vi "Line Configuration Dialog.vi"(8 "error in":errorcluster, 9 "engine configuration in":refnum<class "engine configuration.lvclass">, 10 "tag bus configurable plugin module configuration":refnum<class "DAQmx Module Configuration.lvclass">, 11 "Line":T5={"channel"=refnum, "Physical Channel"="", "Measurement Type"=enum."Digital Input", "Parameters"={"Digital Config"={"Invert Lines?"=FALSE}, "Voltage Config"={"Maximum Value (V)"=5.0, "Minimum Value (V)"=-5.0, "in terminal configuration (V)"=-1, "out terminal configuration (V)"=-1}, "Current Config"={"Maximum Value (A)"=0.02, "Minimum Value (A)"=0.0, "shunt resistor location"=-1, "input terminal configuration (C)"=-1, "external shunt resistor value"=249.0}, "RTD Config"={"Maximum Value (°C)"=100.0, "Minimum Value (°C)"=0.0, "resistance configuration"=2, "r0"=100.0, "current excitation value"=0.0025, "rtd type"=10137, "current excitation source"=10167}, "Thermocouple Config"={"Minimum Value (C)"=0.0, "Maximum Value (C)"=100.0, "thermocouple type"=10072, "cjc source"=10116, "cjc value"=25.0}, "Strain Config"={"Maximum Value"=0.001, "Minimum Value"=-0.001, "bridge information"={"strain configuration"=10183, "lead wire resistance"=0.0, "initial bridge voltage"=0.0, "voltage excitation source"=10200, "voltage excitation value"=2.5}, "strain gage information"={"gage factor"=2.0, "nominal gage resistance"=350.0, "poisson ratio"=0.3}}}} {"Parameters"."Voltage Config"."out terminal configuration (V)" items=["Default"=-1, "RSE"=10083, "Differential"=10106, "Pseudodifferential"=12529]; "Parameters"."Voltage Config"."in terminal configuration (V)" items=["Default"=-1, "RSE"=10083, "NRSE"=10078, "Differential"=10106, "Pseudodifferential"=12529]; "Parameters"."Current Config"."shunt resistor location" items=["default"=-1, "Internal"=10200, "External"=10167]; "Parameters"."Current Config"."input terminal configuration (C)" items=["default"=-1, "RSE"=10083, "NRSE"=10078, "Differential"=10106, "Pseudodifferential"=12529]; "Parameters"."RTD Config"."resistance configuration" items=["2-Wire"=2, "3-Wire"=3, "4-Wire"=4]; "Parameters"."RTD Config"."rtd type" items=["Pt3750"=12481, "Pt3851"=10071, "Pt3911"=12482, "Pt3916"=10069, "Pt3920"=10053, "Pt3928"=12483, "Custom"=10137]; "Parameters"."RTD Config"."current excitation source" items=["Internal"=10200, "External"=10167, "None"=10230]; "Parameters"."Thermocouple Config"."thermocouple type" items=["J"=10072, "K"=10073, "N"=10077, "R"=10082, "S"=10085, "T"=10086, "B"=10047, "E"=10055]; "Parameters"."Thermocouple Config"."cjc source" items=["Built-In"=10200, "Constant Value"=10116, "Channel"=10113]; "Parameters"."Strain Config"."bridge information"."strain configuration" items=["Full Bridge I"=10183, "Full Bridge II"=10184, "Full Bridge III"=10185, "Half Bridge I"=10188, "Half Bridge II"=10189, "Quarter Bridge I"=10271, "Quarter Bridge II"=10272]; "Parameters"."Strain Config"."bridge information"."voltage excitation source" items=["Internal"=10200, "External"=10167, "None"=10230]}) -> (0 "error out":errorcluster, 1 "success":bool, 2 "changed":bool, 3 "Mappings out":T4={"Line"={"channel"=refnum, "Physical Channel"="", "Measurement Type"=enum."Digital Input", "Parameters"={"Digital Config"={"Invert Lines?"=FALSE}, "Voltage Config"={"Maximum Value (V)"=5.0, "Minimum Value (V)"=-5.0, "in terminal configuration (V)"=-1, "out terminal configuration (V)"=-1}, "Current Config"={"Maximum Value (A)"=0.02, "Minimum Value (A)"=0.0, "shunt resistor location"=-1, "input terminal configuration (C)"=-1, "external shunt resistor value"=249.0}, "RTD Config"={"Maximum Value (°C)"=100.0, "Minimum Value (°C)"=0.0, "resistance configuration"=2, "r0"=100.0, "current excitation value"=0.0025, "rtd type"=10137, "current excitation source"=10167}, "Thermocouple Config"={"Minimum Value (C)"=0.0, "Maximum Value (C)"=100.0, "thermocouple type"=10072, "cjc source"=10116, "cjc value"=25.0}, "Strain Config"={"Maximum Value"=0.001, "Minimum Value"=-0.001, "bridge information"={"strain configuration"=10183, "lead wire resistance"=0.0, "initial bridge voltage"=0.0, "voltage excitation source"=10200, "voltage excitation value"=2.5}, "strain gage information"={"gage factor"=2.0, "nominal gage resistance"=350.0, "poisson ratio"=0.3}}}}, "Maps"=[]} {"Line"."Parameters"."Voltage Config"."out terminal configuration (V)" items=["Default"=-1, "RSE"=10083, "Differential"=10106, "Pseudodifferential"=12529]; "Line"."Parameters"."Voltage Config"."in terminal configuration (V)" items=["Default"=-1, "RSE"=10083, "NRSE"=10078, "Differential"=10106, "Pseudodifferential"=12529]; "Line"."Parameters"."Current Config"."shunt resistor location" items=["default"=-1, "Internal"=10200, "External"=10167]; "Line"."Parameters"."Current Config"."input terminal configuration (C)" items=["default"=-1, "RSE"=10083, "NRSE"=10078, "Differential"=10106, "Pseudodifferential"=12529]; "Line"."Parameters"."RTD Config"."resistance configuration" items=["2-Wire"=2, "3-Wire"=3, "4-Wire"=4]; "Line"."Parameters"."RTD Config"."rtd type" items=["Pt3750"=12481, "Pt3851"=10071, "Pt3911"=12482, "Pt3916"=10069, "Pt3920"=10053, "Pt3928"=12483, "Custom"=10137]; "Line"."Parameters"."RTD Config"."current excitation source" items=["Internal"=10200, "External"=10167, "None"=10230]; "Line"."Parameters"."Thermocouple Config"."thermocouple type" items=["J"=10072, "K"=10073, "N"=10077, "R"=10082, "S"=10085, "T"=10086, "B"=10047, "E"=10055]; "Line"."Parameters"."Thermocouple Config"."cjc source" items=["Built-In"=10200, "Constant Value"=10116, "Channel"=10113]; "Line"."Parameters"."Strain Config"."bridge information"."strain configuration" items=["Full Bridge I"=10183, "Full Bridge II"=10184, "Full Bridge III"=10185, "Half Bridge I"=10188, "Half Bridge II"=10189, "Quarter Bridge I"=10271, "Quarter Bridge II"=10272]; "Line"."Parameters"."Strain Config"."bridge information"."voltage excitation source" items=["Internal"=10200, "External"=10167, "None"=10230]})   [LabVIEW 2014, in "DAQmx Module Editor Node.lvclass"]
doc: "A dialog for allowing a user to specify the values of a new line."
uses:
  DAQmx Module Editor Node.lvclass
  module/configuration/Line.ctl
  <vilib>/NI/Tag Bus Module Framework/channel/TBM channel.lvclass
  module/configuration/Measurement Type.ctl
  module/configuration/Parameters.ctl
  Mappings.ctl
  Map.ctl
  <vilib>/NI/Module Execution Interface/Engine Configuration/engine configuration.lvclass
  module/configuration/DAQmx Module Configuration.lvclass
  <vilib>/NI/Tag Bus/tag/tag descriptor.lvclass/tag descriptor.ctl
  <vilib>/NI/Configuration Framework/serializable configuration/NISE_CEF_serializable configuration.lvclass/NISE_CEF_serializable configuration.ctl
  <vilib>/NI/Tag Bus Module Framework/channel/TBM channel.lvclass/TBM channel.ctl
  <vilib>/NI/Tag Bus/tag/write metadata.vi
  <vilib>/NI/Tag Bus/tag/write tag name.vi
  <vilib>/NI/Tag Bus/tag/write data type.vi
  <vilib>/NI/Tag Bus Module Framework/channel/Write channel classification.vi
  <vilib>/NI/Configuration Framework/serializable configuration/Read UID.vi
  <vilib>/NI/Tag Bus/tag/read metadata.vi
  <vilib>/Utility/LVClass/Get LV Class Name.vi
  <vilib>/NI/Configuration Framework/error generator/NISE_error generator.vi
  <vilib>/NI/Tag Bus/tag/tag descriptor.lvclass
  <vilib>/NI/DCAF UI Toolkit/Controls/DCAF UI Elements.lvlib
panel:
  in  "DAQmx Physical Channel":tag
  out "Tab Control":T1(tab)
  in  "Invert Lines?":bool
  in  "out terminal configuration (V)":i32(ring)=-1 items=["Default"=-1, "RSE"=10083, "Differential"=10106, "Pseudodifferential"=12529]
  in  "in terminal configuration (V)":i32(ring)=-1 items=["Default"=-1, "RSE"=10083, "NRSE"=10078, "Differential"=10106, "Pseudodifferential"=12529]
  in  "Maximum Value (V)":dbl=5.0 format="%0.2f"
  in  "Minimum Value (V)":dbl=-5.0 format="%0.2f"
  in  "input terminal configuration (C)":i32(ring)=-1 items=["default"=-1, "RSE"=10083, "NRSE"=10078, "Differential"=10106, "Pseudodifferential"=12529]
  in  "shunt resistor location":i32(ring)=-1 items=["default"=-1, "Internal"=10200, "External"=10167]
  in  "external shunt resistor value":dbl=249.0 format="%0.2f"
  in  "Maximum Value (A)":dbl=0.02 format="%0.5f"
  in  "Minimum Value (A)":dbl format="%0.5f"
  in  "r0":dbl=100.0 format="%0.2f"
  in  "resistance configuration":i32(ring)=2 items=["2-Wire"=2, "3-Wire"=3, "4-Wire"=4]
  in  "Maximum Value (°C)":dbl=100.0 format="%0.2f"
  in  "Minimum Value (°C)":dbl format="%0.2f"
  in  "rtd type":i32(ring)=12481 items=["Pt3750"=12481, "Pt3851"=10071, "Pt3911"=12482, "Pt3916"=10069, "Pt3920"=10053, "Pt3928"=12483, "Custom"=10137]
  in  "current excitation value":dbl=0.0025 format="%0.5f"
  in  "current excitation source":i32(ring)=10167 items=["Internal"=10200, "External"=10167, "None"=10230]
  in  "strain gage information":T2={"gage factor"=2.0, "nominal gage resistance"=350.0, "poisson ratio"=0.3} {"poisson ratio" format="%0.2f"; "nominal gage resistance" format="%0.2f"; "gage factor" format="%0.2f"}
  in  "bridge information":T3={"strain configuration"=10183, "lead wire resistance"=0.0, "initial bridge voltage"=0.0, "voltage excitation source"=10200, "voltage excitation value"=2.5} {"initial bridge voltage" format="%0.2f"; "voltage excitation source" items=["Internal"=10200, "External"=10167, "None"=10230]; "voltage excitation value" format="%0.2f"; "lead wire resistance" format="%0.2f"; "strain configuration" items=["Full Bridge I"=10183, "Full Bridge II"=10184, "Full Bridge III"=10185, "Half Bridge I"=10188, "Half Bridge II"=10189, "Quarter Bridge I"=10271, "Quarter Bridge II"=10272]}
  in  "Minimum Value":dbl=-0.001 format="%0.7f"
  in  "Maximum Value":dbl=0.001 format="%0.7f"
  in  "cjc value":dbl=25.0 format="%0.2f"
  in  "thermocouple type":i32(ring)=10072 items=["J"=10072, "K"=10073, "N"=10077, "R"=10082, "S"=10085, "T"=10086, "B"=10047, "E"=10055]
  in  "Maximum Value (C)":dbl=100.0 format="%0.2f"
  in  "Minimum Value (C)":dbl format="%0.2f"
  in  "cjc source":i32(ring)=10116 items=["Built-In"=10200, "Constant Value"=10116, "Channel"=10113]
  in  "Measurement Type":i32(listbox)
  out "errors":string
  in  "Tag":i32(listbox)
  in  "Description":string
  in  "cancel":bool
  in  "ok":bool
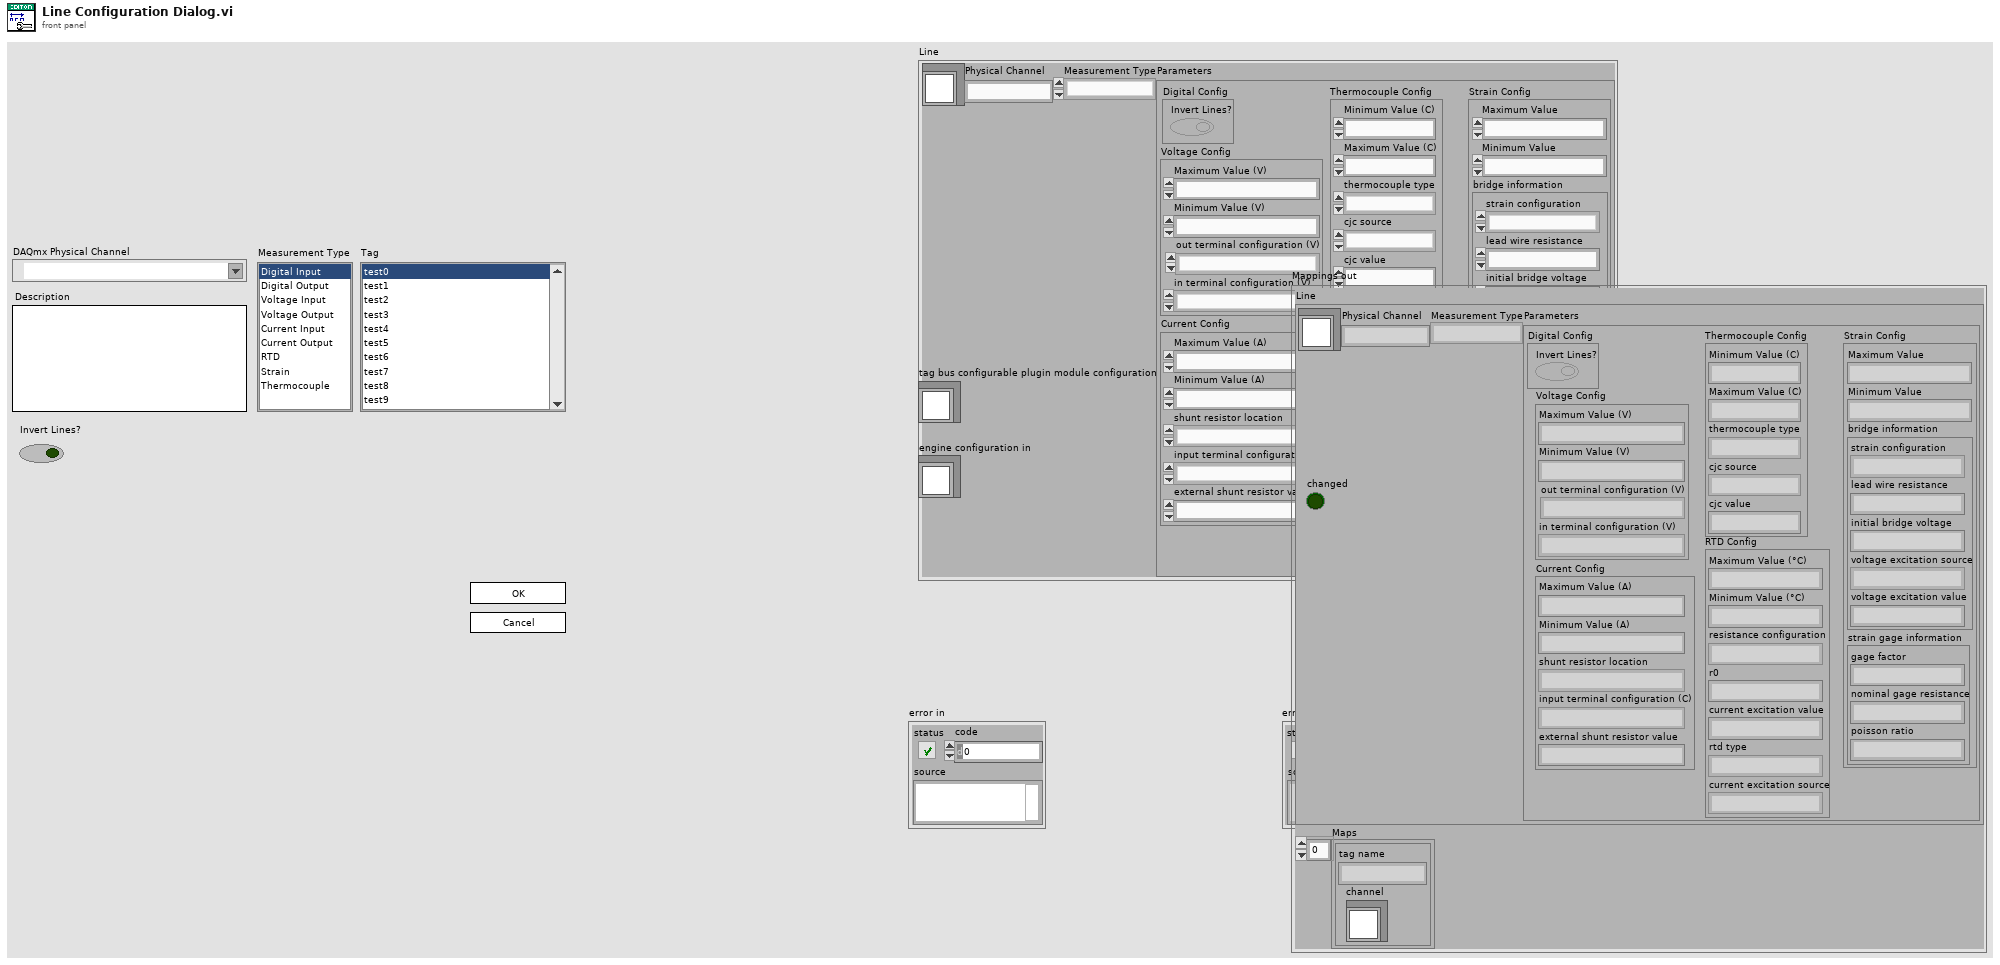
[diagram p1: front panel]
types:
  T1 = enum32{"Digital", "Voltage", "Current", "RTD", "Strain", "Thermocouple"}
  T2 = cluster{"gage factor":dbl, "nominal gage resistance":dbl, "poisson ratio":dbl}
  T3 = cluster{"strain configuration":i32, "lead wire resistance":dbl, "initial bridge voltage":dbl, "voltage excitation source":i32, "voltage excitation value":dbl}
  T4 = typedef "DAQmx Module Editor Node.lvclass/Mappings.ctl" = cluster{"Line":T5, "Maps":T8[]}
  T5 = typedef "DAQmx Module Configuration.lvclass/Line.ctl" = cluster{"channel":refnum<class "TBM channel.lvclass">, "Physical Channel":string, "Measurement Type":T6, "Parameters":T7}
  T6 = typedef "DAQmx Module Configuration.lvclass/Measurement Type.ctl" = enum16{"Digital Input", "Digital Output", "Voltage Input", "Voltage Output", "Current Input", "Current Output", "RTD", "Thermocouple", "Strain"}
  T7 = typedef "DAQmx Module Configuration.lvclass/Parameters.ctl" = cluster{"Digital Config":cluster{"Invert Lines?":bool}, "Voltage Config":cluster{"Maximum Value (V)":dbl, "Minimum Value (V)":dbl, "in terminal configuration (V)":i32, "out terminal configuration (V)":i32}, "Current Config":cluster{"Maximum Value (A)":dbl, "Minimum Value (A)":dbl, "shunt resistor location":i32, "input terminal configuration (C)":i32, "external shunt resistor value":dbl}, "RTD Config":cluster{"Maximum Value (°C)":dbl, "Minimum Value (°C)":dbl, "resistance configuration":i32, "r0":dbl, "current excitation value":dbl, "rtd type":i32, "current excitation source":i32}, "Thermocouple Config":cluster{"Minimum Value (C)":dbl, "Maximum Value (C)":dbl, "thermocouple type":i32, "cjc source":i32, "cjc value":dbl}, "Strain Config":cluster{"Maximum Value":dbl, "Minimum Value":dbl, "bridge information":cluster{"strain configuration":i32, "lead wire resistance":dbl, "initial bridge voltage":dbl, "voltage excitation source":i32, "voltage excitation value":dbl}, "strain gage information":cluster{"gage factor":dbl, "nominal gage resistance":dbl, "poisson ratio":dbl}}}
  T8 = typedef "Daqmx Module editor node.lvclass/Map.ctl" = cluster{"channel":refnum<class "TBM channel.lvclass">, "tag name":string}
  T9 = typedef "Daqmx Module configuration.lvclass/Measurement Type.ctl" = enum16{"Digital Input", "Digital Output", "Voltage Input", "Voltage Output", "Current Input", "Current Output", "RTD", "Thermocouple", "Strain"}
  T10 = enum8{"Enabled", "Disabled", "Disabled and Grayed Out"}
  T11 = typedef "TBM channel.lvclass/channel classification.ctl" = enum16{"input data", "output data", "processing parameter", "processing result"}
  T12 = typedef "tag bus.lvlib/tag descriptor.lvclass/Data Type.ctl" = enum16{"Double", "Single", "I64", "I32", "I16", "I8", "U64", "U32", "U16", "U8", "Boolean", "String", "Array of Double", "Array of Single", "Array of I64", "Array of I32", "Array of I16", "Array of I8", "Array of U64", "Array of U32", "Array of U16", "Array of U8", "Array of Boolean", "Array of String"}
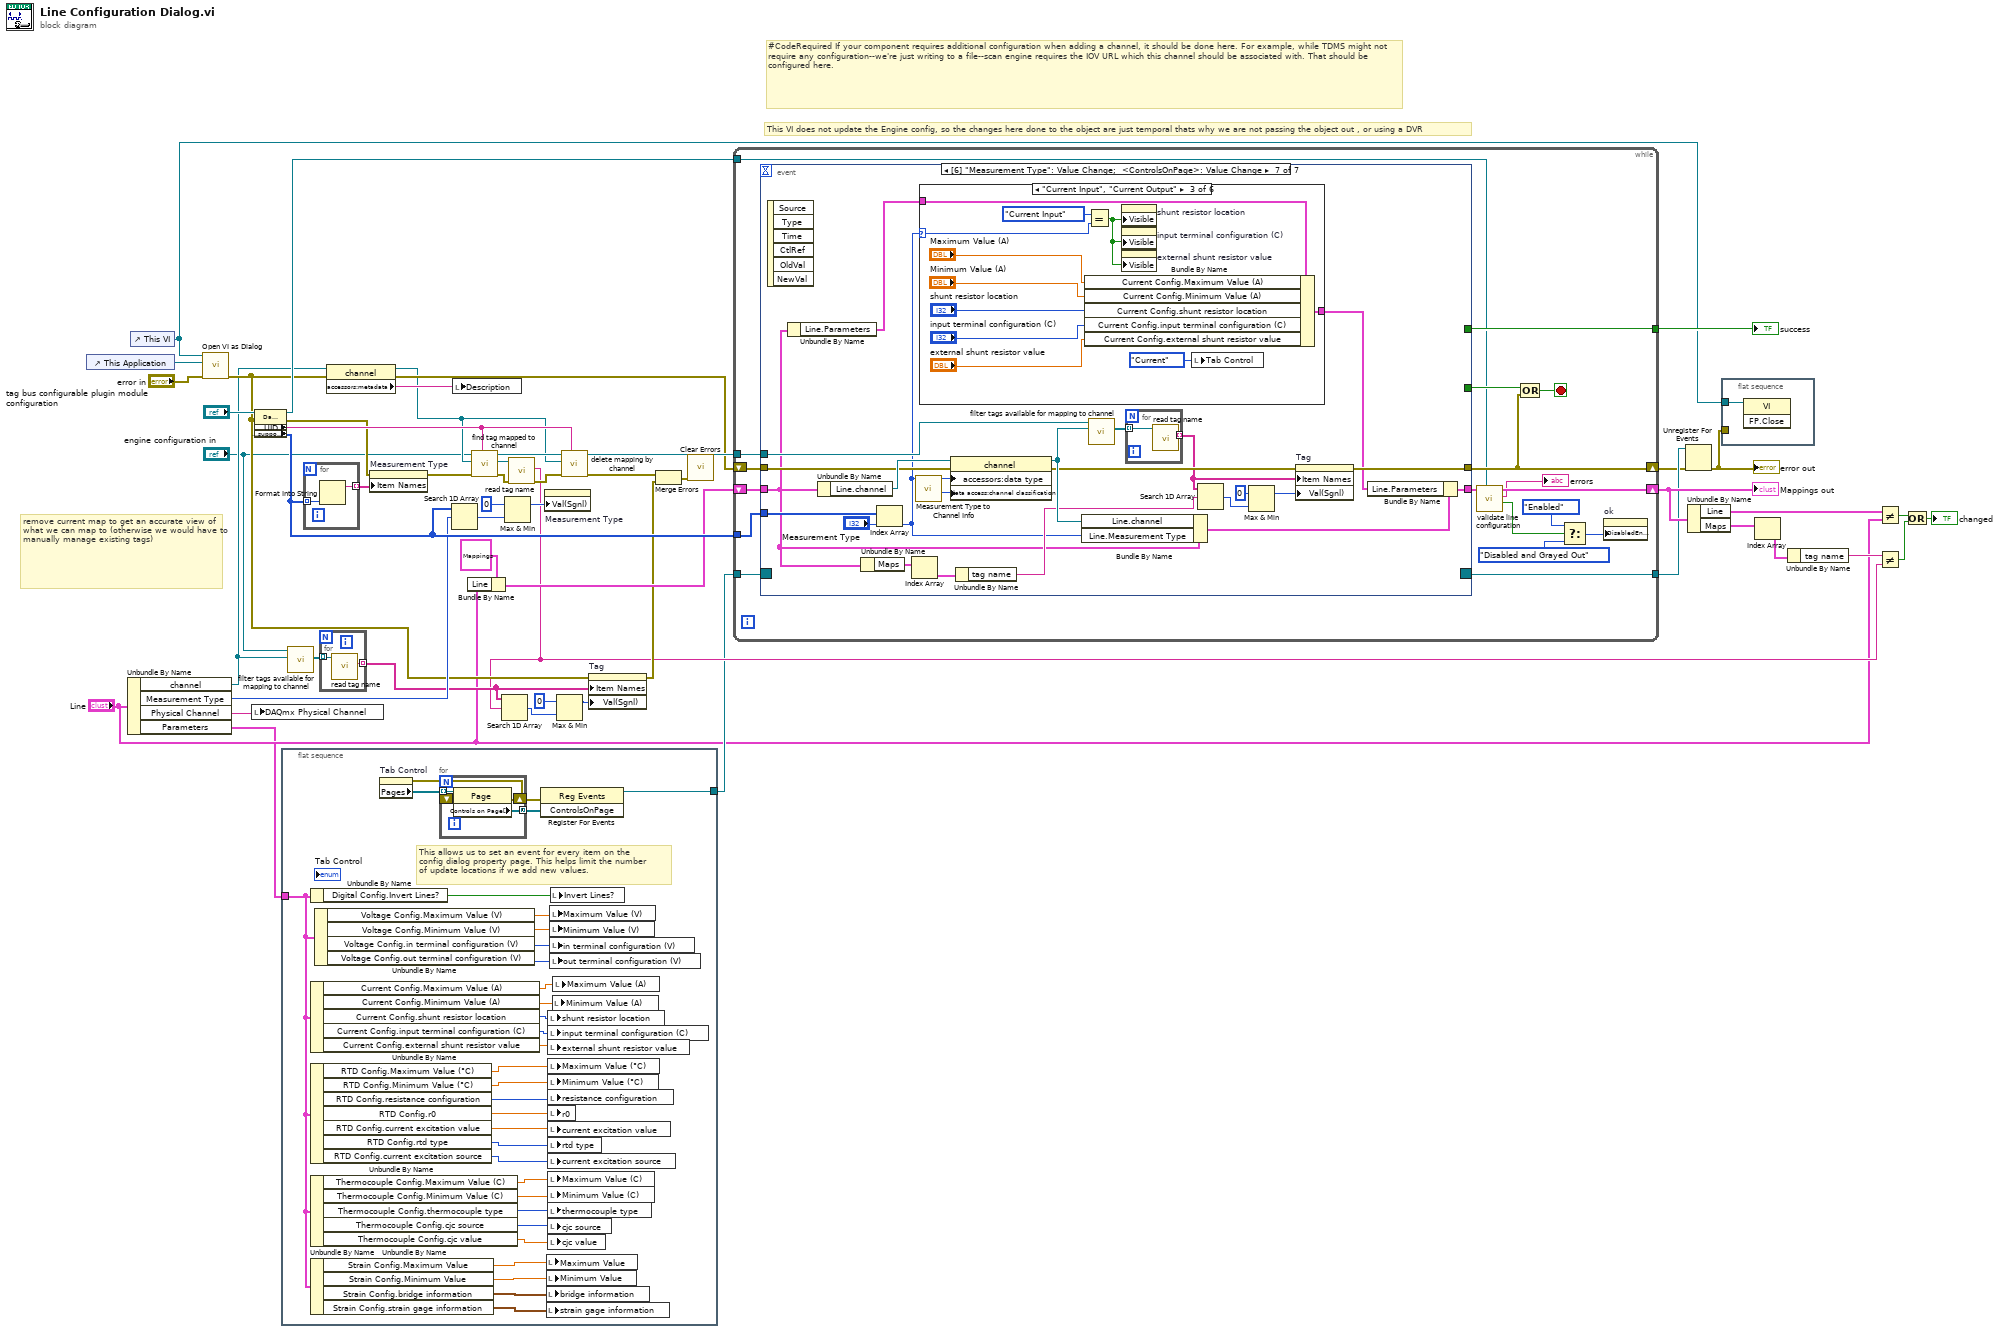
[diagram p0: block diagram]
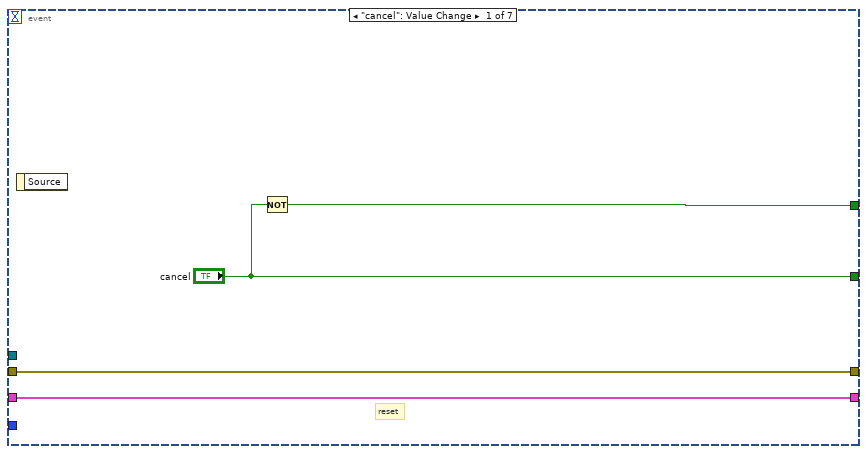
[diagram p2: hidden frame]
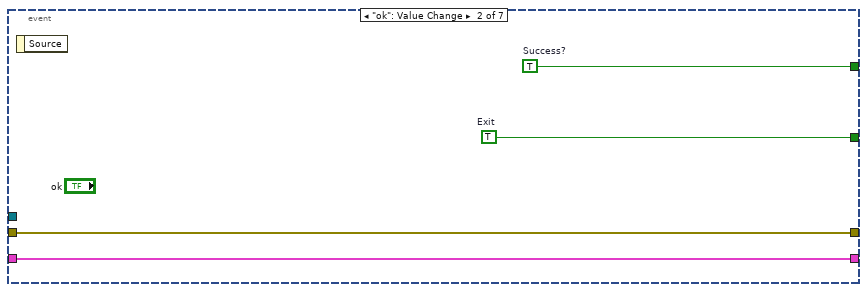
[diagram p3: hidden frame]
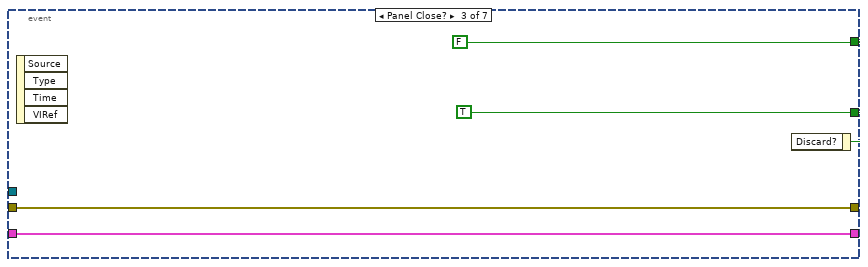
[diagram p4: hidden frame]
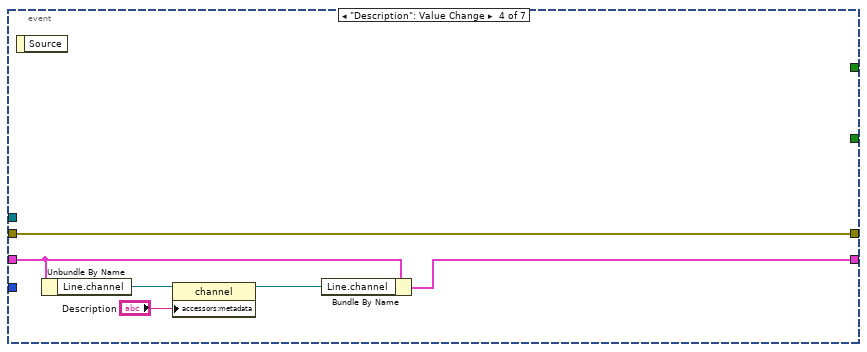
[diagram p5: hidden frame]
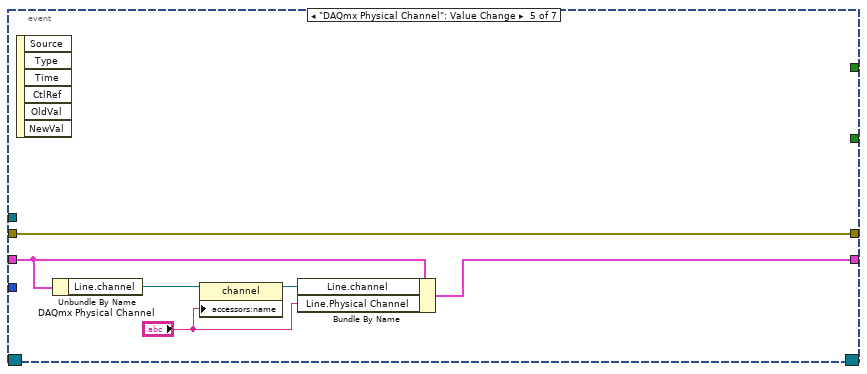
[diagram p6: hidden frame]
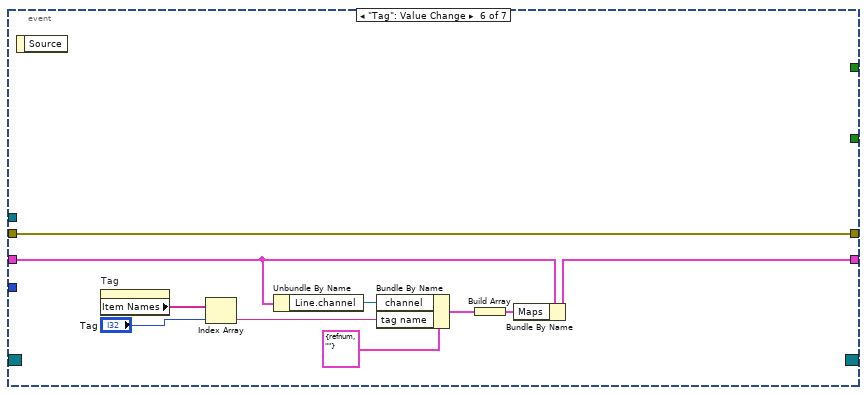
[diagram p7: hidden frame]
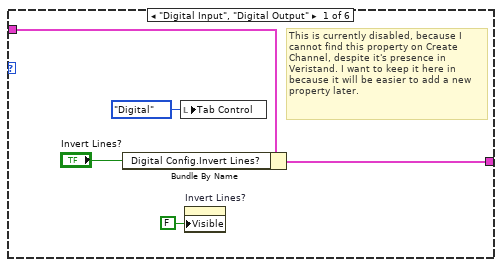
[diagram p8: hidden frame]
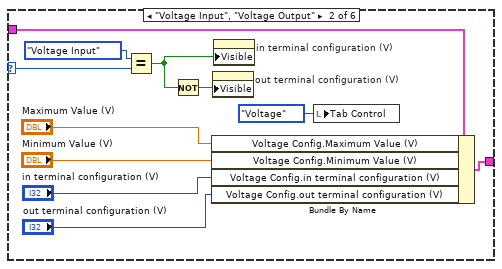
[diagram p9: hidden frame]
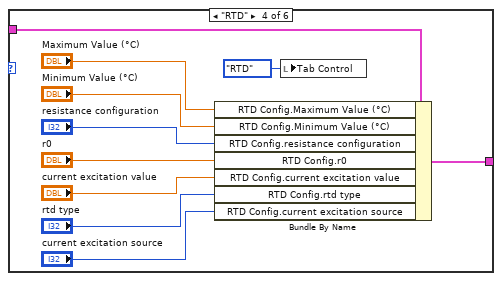
[diagram p10: hidden frame]
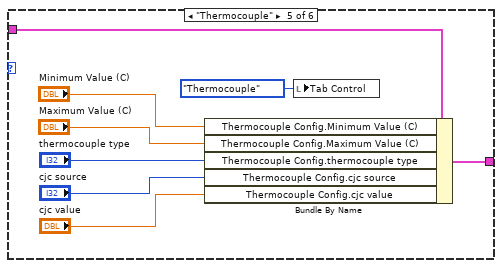
[diagram p11: hidden frame]
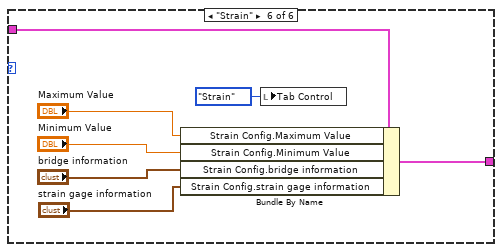
[diagram p12: hidden frame]
diagram:
  # "This VI does not update the Engine config, so the changes here done to the object are just temporal thats why we are not passing the object out , or using a DVR"
  # "remove current map to get an accurate view of what we can map to (otherwise we would have to manually manage existing tags)"
  # "#CodeRequired If your component requires additional configuration when adding a channel, it should be done here. For example, while TDMS might not require any configuration--we're just writing to a file--scan engine requires the IOV URL which this channel should be associated with. That should be configured here."
  n1 = control-ref of="This Application"() -> (w45:refnum<vi>)
  n2 = Unbundle By Name("Line") -> ("channel"=w17:refnum<class "TBM channel.lvclass">, "Measurement Type"=w22:T6, "Physical Channel"=w21:string, "Parameters"=w5:T7)
  n3 = control-ref of="This VI"() -> (w29:refnum<vi>)
  n4 = call <vilib>:"Open VI as Dialog.vi"("error in (no error)"="error in", "This Application"=w45, "VI in"=w29) -> ("error out"=w18:errorcluster)  [unwired: 8 in]
  n5 = local write "DAQmx Physical Channel"(w21) -> ()
  n6 = property class="Daqmx Module configuration"(reference="tag bus configurable plugin module configuration", error in=w18) -> (reference out=w40:refnum<class "DAQmx Module Configuration.lvclass">, error out=w27:errorcluster, "Properties:UID"=w43:string, "Customize:Properties:supported measurement types"=w23:T9[])
  n7 = flat-sequence {
    tunnel: [w84] -> w7
    tunnel: w5 -> [w58]
    frame #0 {
      # "This allows us to set an event for every item on the \nconfig dialog property page. This helps limit the number \nof update locations if we add new values."
      n8 = Unbundle By Name(w58) -> ("Digital Config.Invert Lines?"=w79:bool)
      n9 = Unbundle By Name(w58) -> ("Current Config.Maximum Value (A)"=w71:dbl, "Current Config.Minimum Value (A)"=w72:dbl, "Current Config.shunt resistor location"=w74:i32, "Current Config.input terminal configuration (C)"=w83:i32, "Current Config.external shunt resistor value"=w73:dbl)
      n10 = Unbundle By Name(w58) -> ("RTD Config.Maximum Value (°C)"=w70:dbl, "RTD Config.Minimum Value (°C)"=w69:dbl, "RTD Config.resistance configuration"=w68:i32, "RTD Config.r0"=w67:dbl, "RTD Config.current excitation value"=w66:dbl, "RTD Config.rtd type"=w65:i32, "RTD Config.current excitation source"=w64:i32)
      n11 = Unbundle By Name(w58) -> ("Thermocouple Config.Maximum Value (C)"=w61:dbl, "Thermocouple Config.Minimum Value (C)"=w62:dbl, "Thermocouple Config.thermocouple type"=w63:i32, "Thermocouple Config.cjc source"=w60:i32, "Thermocouple Config.cjc value"=w59:dbl)
      n12 = Unbundle By Name(w58) -> ("Strain Config.Maximum Value"=w75:dbl, "Strain Config.Minimum Value"=w76:dbl, "Strain Config.bridge information"=w77:T3, "Strain Config.strain gage information"=w78:T2)
      n13 = Unbundle By Name(w58) -> ("Voltage Config.Maximum Value (V)"=w82:dbl, "Voltage Config.Minimum Value (V)"=w81:dbl, "Voltage Config.in terminal configuration (V)"=w80:i32, "Voltage Config.out terminal configuration (V)"=w57:i32)
      n14 = property on="Tab Control" class="TabCtl (strict)"() -> (error out=w55:errorcluster, "Pages"=w56:refnum<vi>[])  [unwired: 2 in, 1 out]
      n15 = for {
        tunnel: w56 -> [w88] mode=indexing
        tunnel: [w85] -> w53 mode=concatenating
        shift-right: [w86] -> w54
        shift-left: w55 -> [w87]
        n16 = property class="Page"(reference=w88, error in=w87) -> (error out=w86:errorcluster, "Controls on Page[]"=w85:refnum<vi>[])  [unwired: 1 out]
      }
      n17 = register-events(error in=w54, w53) -> (reference out=w84:refnum<event-registration>)  [unwired: 1 in, 1 out]
      n18 = local write "Maximum Value"(w75) -> ()
      n19 = local write "Minimum Value"(w76) -> ()
      n20 = local write "bridge information"(w77) -> ()
      n21 = local write "strain gage information"(w78) -> ()
      n22 = local write "shunt resistor location"(w74) -> ()
      n23 = local write "input terminal configuration (C)"(w83) -> ()
      n24 = local write "external shunt resistor value"(w73) -> ()
      n25 = local write "Maximum Value (°C)"(w70) -> ()
      n26 = local write "Minimum Value (°C)"(w69) -> ()
      n27 = local write "resistance configuration"(w68) -> ()
      n28 = local write "r0"(w67) -> ()
      n29 = local write "current excitation value"(w66) -> ()
      n30 = local write "rtd type"(w65) -> ()
      n31 = local write "current excitation source"(w64) -> ()
      n32 = local write "Maximum Value (C)"(w61) -> ()
      n33 = local write "Minimum Value (C)"(w62) -> ()
      n34 = local write "thermocouple type"(w63) -> ()
      n35 = local write "cjc source"(w60) -> ()
      n36 = local write "cjc value"(w59) -> ()
      n37 = local write "Maximum Value (V)"(w82) -> ()
      n38 = local write "Minimum Value (V)"(w81) -> ()
      n39 = local write "in terminal configuration (V)"(w80) -> ()
      n40 = local write "out terminal configuration (V)"(w57) -> ()
      n41 = local write "Invert Lines?"(w79) -> ()
      n42 = local write "Minimum Value (A)"(w72) -> ()
      n43 = local write "Maximum Value (A)"(w71) -> ()
    }
  }
  n44 = call-dynamic "filter tags available for mapping to channel.vi"("channel to map to"=w17, "engine configuration in"="engine configuration in") -> ("filtered tags"=w19:refnum<class "tag descriptor.lvclass">[])  [unwired: 8 in, 1 out]
  n45 = for {
    tunnel: w23 -> [w90] mode=indexing
    tunnel: [w89] -> w28 mode=indexing
    n46 = Format Into String(w90) -> (resulting string=w89:string)  [unwired: 3 in, 1 out]
  }
  n47 = for {
    tunnel: w19 -> [w92] mode=indexing
    tunnel: [w91] -> w15 mode=indexing
    n48 = call <vilib>:"read tag name.vi"("system tag in"=w92) -> ("name"=w91:string)  [unwired: 8 in, 2 out]
  }
  n49 = property class="channel"(reference=w17, error in=w18) -> (reference out=w39:refnum<class "TBM channel.lvclass">, error out=w41:errorcluster, "accessors:metadata"=w50:string)
  n50 = property on="Measurement Type" class="LstBox (strict)"(error in=w27, "Item Names"=w28) -> (error out=w1:errorcluster)  [unwired: 1 in, 1 out]
  n51 = Search 1D Array(1D array=w23, element=w22) -> (index of element=w24:i32)  [unwired: 1 in]
  n52 = local write "Description"(w50) -> ()
  n53 = Bundle By Name(cluster=T4 {"Line"={"channel"=refnum, "Physical Channel"="", "Measurement Type"=enum."Digital Input", "Parameters"={"Digital Config"={"Invert Lines?"=FALSE}, "Voltage Config"={"Maximum Value (V)"=5.0, "Minimum Value (V)"=-5.0, "in terminal configuration (V)"=-1, "out terminal configuration (V)"=-1}, "Current Config"={"Maximum Value (A)"=0.02, "Minimum Value (A)"=0.0, "shunt resistor location"=-1, "input terminal configuration (C)"=-1, "external shunt resistor value"=249.0}, "RTD Config"={"Maximum Value (°C)"=100.0, "Minimum Value (°C)"=0.0, "resistance configuration"=2, "r0"=100.0, "current excitation value"=0.0025, "rtd type"=10137, "current excitation source"=10167}, "Thermocouple Config"={"Minimum Value (C)"=0.0, "Maximum Value (C)"=100.0, "thermocouple type"=10072, "cjc source"=10116, "cjc value"=25.0}, "Strain Config"={"Maximum Value"=0.001, "Minimum Value"=-0.001, "bridge information"={"strain configuration"=10183, "lead wire resistance"=0.0, "initial bridge voltage"=0.0, "voltage excitation source"=10200, "voltage excitation value"=2.5}, "strain gage information"={"gage factor"=2.0, "nominal gage resistance"=350.0, "poisson ratio"=0.3}}}}, "Maps"=[]} ("Mappings out"), "Line"="Line") -> (w20:T4)
  n54 = call <vilib>:"find tag mapped to channel.vi"("owner"=w43, "error in"=w1, "channel"=w39, "engine configuration in"="engine configuration in") -> ("error out"=w37:errorcluster, "tag"=w38:refnum<class "tag descriptor.lvclass">, "engine configuration out"=w42:refnum<class "engine configuration.lvclass">)  [unwired: 5 in]
  n55 = Max & Min(x=0 ("f"), y=w24) -> (max(x,y)=w26:i32)  [unwired: 1 out]
  n56 = call <vilib>:"read tag name.vi"("error in"=w37, "system tag in"=w38) -> ("error out"=w36:errorcluster, "name"=w9:string)  [unwired: 7 in, 1 out]
  n57 = Search 1D Array(1D array=w15, element=w9) -> (index of element=w10:i32)  [unwired: 1 in]
  n58 = property on="Measurement Type" class="LstBox (strict)"("Val(Sgnl)"=w26) -> ()  [unwired: 2 in, 2 out]
  n59 = Max & Min(x=0 ("f"), y=w10) -> (max(x,y)=w8:i32)  [unwired: 1 out]
  n60 = call <vilib>:"delete mapping by channel.vi"("owner ID"=w43, "error in"=w36, "channel"=w39, "engine configuration in"=w42) -> ("error out"=w14:errorcluster, "engine configuration out"=w51:refnum<class "engine configuration.lvclass">)  [unwired: 6 in]
  n61 = property on="Tag" class="LstBox (strict)"(error in=w18, "Item Names"=w15, "Val(Sgnl)"=w8) -> (error out=w13:errorcluster)  [unwired: 1 in, 1 out]
  n62 = Merge Errors(w14, w13) -> (w12:errorcluster)
  n63 = call <vilib>:"Clear Errors.vi"("error in (no error)"=w12) -> ()  [unwired: 5 in, 2 out]
  n64 = while {
    shift-right: [w102] -> w3
    shift-left: w41 -> [w109]
    tunnel: [w108] -> w52
    shift-right: [w103] -> w46
    shift-left: w20 -> [w105]
    tunnel: w51 -> [w110]
    tunnel: w40 -> [w94]
    tunnel: w23 -> [w96]
    tunnel: w7 -> [w95]
    tunnel: [w93] -> w4
    stop <- w106 stop-if-true
    n65 = event shown="[6] \"Measurement Type\": Value Change;  <ControlsOnPage>: Value Change" {
      selector: w95 -> [_ _ _ _ _ _ _]
      dyn-events: [_ _ _ _ _ _ _] -> w93
      timeout: _ -> [_ _ _ _ _ _ _]
      tunnel: w110 -> [_ _ _ _ _ _ w159]
      tunnel: w109 -> [w114 w118 w122 w128 w134 w144 w165]
      tunnel: [w114 w118 w122 w128 w134 w144 w163] -> w102
      tunnel: [w113 w115 FALSE _ _ _ _] -> w108
      tunnel: ["cancel" w116 w120 _ _ _ _] -> w107
      tunnel: w105 -> [w111 w117 w119 w126 w132 w139 w151]
      tunnel: [w111 w117 w119 w127 w133 w136 w149] -> w104
      tunnel: w96 -> [_ _ _ _ _ _ w157]
      event "cancel": Value Change {
        # "reset"
        n66 = event-data() -> ()  [unwired: 1 in, 1 out]
        n67 = Not(x="cancel") -> (.not. x?=w113:bool)
      }
      event "ok": Value Change {
        w115 = TRUE  # Success?
        w116 = TRUE  # Exit
        n68 = event-data() -> ()  [unwired: 1 in, 1 out]
      }
      event Panel Close? {
        w120 = TRUE ("cancel")
        n69 = event-data() -> ()  [unwired: 1 in, 4 out]
        n70 = event-data("Discard?"=w120) -> ()  [unwired: 1 in, 1 out]
      }
      event "Description": Value Change {
        n71 = event-data() -> ()  [unwired: 1 in, 1 out]
        n72 = Unbundle By Name(w126) -> ("Line.channel"=w125:refnum<class "TBM channel.lvclass">)
        n73 = property class="channel"(reference=w125, "accessors:metadata"="Description") -> (reference out=w124:refnum<class "TBM channel.lvclass">)  [unwired: 1 in, 1 out]
        n74 = Bundle By Name(cluster=w126, "Line.channel"=w124) -> (w127:T4)
      }
      event "DAQmx Physical Channel": Value Change {
        n75 = event-data() -> ()  [unwired: 1 in, 6 out]
        n76 = Unbundle By Name(w132) -> ("Line.channel"=w131:refnum<class "TBM channel.lvclass">)
        n77 = property class="channel"(reference=w131, "accessors:name"="DAQmx Physical Channel") -> (reference out=w130:refnum<class "TBM channel.lvclass">)  [unwired: 1 in, 1 out]
        n78 = Bundle By Name(cluster=w132, "Line.channel"=w130, "Line.Physical Channel"="DAQmx Physical Channel") -> (w133:T4)
      }
      event "Tag": Value Change {
        n79 = event-data() -> ()  [unwired: 1 in, 1 out]
        n80 = property on="Tag" class="LstBox (strict)"() -> ("Item Names"=w142:string[])  [unwired: 2 in, 2 out]
        n81 = Index Array(array=w142, index="Tag") -> (element=w135:string)
        n82 = Unbundle By Name(w139) -> ("Line.channel"=w140:refnum<class "TBM channel.lvclass">)
        n83 = Bundle By Name(cluster=T8 {"channel"=refnum, "tag name"=""} ("Map"), "channel"=w140, "tag name"=w135) -> (w138:T8)
        n84 = Build Array(w138) -> (w137:T8[])
        n85 = Bundle By Name(cluster=w139, "Maps"=w137) -> (w136:T4)
      }
      event "Measurement Type": Value Change {
        n86 = event-data() -> ()  [unwired: 1 in, 6 out]
        n87 = Unbundle By Name(w151) -> ("Line.Parameters"=w148:T7)
        n88 = Unbundle By Name(w151) -> ("Line.channel"=w168:refnum<class "TBM channel.lvclass">)
        n89 = Unbundle By Name(w151) -> ("Maps"=w161:T8[])
        n90 = Index Array(array=w157, index="Measurement Type") -> (element=w152:T9)
        n91 = Index Array(array=w161) -> (element=w160:T8)  [unwired: 1 in]
        n92 = call "Measurement Type to Channel Info.vi"("Measurement Type"=w152) -> ("channel classification"=w145:T11, "Data Type"=w146:T12)  [unwired: 8 in]
        n93 = case shown="\"Current Input\", \"Current Output\"" w152 {
          selector: w152 -> [_ w183 w186 _ _ _]
          tunnel: [w171 w179 w187 w197 w207 w215] -> w147
          tunnel: w148 -> [w170 w177 w185 w196 w206 w214]
          frame "Digital Input", "Digital Output" {
            # "This is currently disabled, because I \ncannot find this property on Create\nChannel, despite it's presence in\nVeristand. I want to keep it here in \nbecause it will be easier to add a new \nproperty later."
            n94 = Bundle By Name(cluster=w170, "Digital Config.Invert Lines?"="Invert Lines?") -> (w171:T7)
            n95 = local write "Tab Control"(T1."Digital" ("Tab Control")) -> ()
            n96 = property on="Invert Lines?" class="Bool (strict)"("Visible"=FALSE) -> ()  [unwired: 2 in, 2 out]
          }
          frame "Voltage Input", "Voltage Output" {
            n97 = Equal?(x=Measurement_Type."Voltage Input", y=w183) -> (x = y?=w174:bool)
            n98 = Not(x=w174) -> (.not. x?=w175:bool)
            n99 = Bundle By Name(cluster=w177, "Voltage Config.Maximum Value (V)"="Maximum Value (V)", "Voltage Config.Minimum Value (V)"="Minimum Value (V)", "Voltage Config.in terminal configuration (V)"="in terminal configuration (V)", "Voltage Config.out terminal configuration (V)"="out terminal configuration (V)") -> (w179:T7)
            n100 = property on="out terminal configuration (V)" class="Ring (strict)"("Visible"=w175) -> ()  [unwired: 2 in, 2 out]
            n101 = property on="in terminal configuration (V)" class="Ring (strict)"("Visible"=w174) -> ()  [unwired: 2 in, 2 out]
            n102 = local write "Tab Control"(T1."Voltage" ("Tab Control")) -> ()
          }
          frame "Current Input", "Current Output" {
            n103 = Bundle By Name(cluster=w185, "Current Config.Maximum Value (A)"="Maximum Value (A)", "Current Config.Minimum Value (A)"="Minimum Value (A)", "Current Config.shunt resistor location"="shunt resistor location", "Current Config.input terminal configuration (C)"="input terminal configuration (C)", "Current Config.external shunt resistor value"="external shunt resistor value") -> (w187:T7)
            n104 = Equal?(x=Measurement_Type."Current Input", y=w186) -> (x = y?=w194:bool)
            n105 = property on="shunt resistor location" class="Ring (strict)"("Visible"=w194) -> ()  [unwired: 2 in, 2 out]
            n106 = property on="input terminal configuration (C)" class="Ring (strict)"("Visible"=w194) -> ()  [unwired: 2 in, 2 out]
            n107 = property on="external shunt resistor value" class="DigNum (strict)"("Visible"=w194) -> ()  [unwired: 2 in, 2 out]
            n108 = local write "Tab Control"(T1."Current" ("Tab Control")) -> ()
          }
          frame "RTD" {
            n109 = Bundle By Name(cluster=w196, "RTD Config.Maximum Value (°C)"="Maximum Value (°C)", "RTD Config.Minimum Value (°C)"="Minimum Value (°C)", "RTD Config.resistance configuration"="resistance configuration", "RTD Config.r0"="r0", "RTD Config.current excitation value"="current excitation value", "RTD Config.rtd type"="rtd type", "RTD Config.current excitation source"="current excitation source") -> (w197:T7)
            n110 = local write "Tab Control"(T1."RTD" ("Tab Control")) -> ()
          }
          frame "Thermocouple" {
            n111 = Bundle By Name(cluster=w206, "Thermocouple Config.Minimum Value (C)"="Minimum Value (C)", "Thermocouple Config.Maximum Value (C)"="Maximum Value (C)", "Thermocouple Config.thermocouple type"="thermocouple type", "Thermocouple Config.cjc source"="cjc source", "Thermocouple Config.cjc value"="cjc value") -> (w207:T7)
            n112 = local write "Tab Control"(T1."Thermocouple" ("Tab Control")) -> ()
          }
          frame "Strain" {
            n113 = Bundle By Name(cluster=w214, "Strain Config.Maximum Value"="Maximum Value", "Strain Config.Minimum Value"="Minimum Value", "Strain Config.bridge information"="bridge information", "Strain Config.strain gage information"="strain gage information") -> (w215:T7)
            n114 = local write "Tab Control"(T1."Strain" ("Tab Control")) -> ()
          }
        }
        n115 = property class="channel"(reference=w168, error in=w165, "accessors:data type"=w146, "data access:channel classification"=w145) -> (reference out=w167:refnum<class "TBM channel.lvclass">, error out=w164:errorcluster)
        n116 = Unbundle By Name(w160) -> ("tag name"=w155:string)
        n117 = Bundle By Name(cluster=w151, "Line.channel"=w167, "Line.Measurement Type"=w152) -> (w150:T4)
        n118 = call-dynamic "filter tags available for mapping to channel.vi"("channel to map to"=w167, "engine configuration in"=w159) -> ("filtered tags"=w166:refnum<class "tag descriptor.lvclass">[])  [unwired: 8 in, 1 out]
        n119 = for {
          tunnel: w166 -> [w222] mode=indexing
          tunnel: [w221] -> w162 mode=indexing
          n120 = call <vilib>:"read tag name.vi"("system tag in"=w222) -> ("name"=w221:string)  [unwired: 8 in, 2 out]
        }
        n121 = Search 1D Array(1D array=w162, element=w155) -> (index of element=w153:i32)  [unwired: 1 in]
        n122 = Max & Min(x=0 ("f"), y=w153) -> (max(x,y)=w154:i32)  [unwired: 1 out]
        n123 = property on="Tag" class="LstBox (strict)"(error in=w164, "Item Names"=w162, "Val(Sgnl)"=w154) -> (error out=w163:errorcluster)  [unwired: 1 in, 1 out]
        n124 = Bundle By Name(cluster=w150, "Line.Parameters"=w147) -> (w149:T4)
      }
    }
    n125 = call "validate line configuration.vi"("Module Config"=w94, "Mappings in"=w104) -> ("valid?"=w101:bool, "errors"=→"errors":string, "Mappings out"=w103:T4)  [unwired: 7 in]
    n126 = Compound Arithmetic op=OR(w107, w102) -> (w106:bool)
    n127 = Select(t=T10."Enabled" ("Disabled"), s=w101, f=T10."Disabled and Grayed Out") -> (s? t:f=w98:T10)
    n128 = property on="ok" class="Bool"("DisabledEnum"=w98) -> ()  [unwired: 2 in, 2 out]
  }
  "success" <- w52
  "Mappings out" <- w46
  n129 = Unregister For Events(event registration refnum=w4, error in=w3) -> (error out=w2:errorcluster)
  "error out" <- w2
  n130 = Unbundle By Name(w46) -> ("Line"=w47:T5, "Maps"=w35:T8[])
  n131 = flat-sequence {
    tunnel: w2 -> [_]
    tunnel: w29 -> [w223]
    frame #0 {
      n132 = invoke class="VI" method="FP.Close"(reference=w223) -> ()  [unwired: 2 in, 3 out]
    }
  }
  n133 = Index Array(array=w35) -> (element=w34:T8)  [unwired: 1 in]
  n134 = Unbundle By Name(w34) -> ("tag name"=w33:string)
  n135 = Not Equal?(x=w47, y="Line") -> (x != y?=w31:bool)
  n136 = Not Equal?(x=w33, y=w9) -> (x != y?=w32:bool)
  n137 = Or(x=w31, y=w32) -> (x .or. y?=→"changed":bool)
